vi "Toolkit Error Handling - Add Caller to API VI List.vi"(8 "error in":errorcluster) -> (0 "error out":errorcluster)   [LabVIEW 2011]
doc: "Add this VI's caller to the Toolkit API list. This is used by the Toolkit Error Handling framework to hide the call-chain of low-level support VIs."
panel:
  # "THIS VI MUST BE REENTRANT"
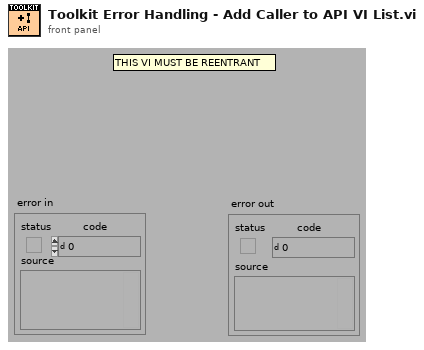
[diagram p1: front panel]
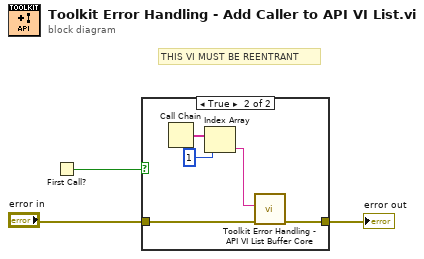
[diagram p0: block diagram]
diagram:
  # "THIS VI MUST BE REENTRANT"
  n1 = First Call?() -> (First Call?: T/F=w1:bool)
  n2 = case shown="True" w1 {
    tunnel: [w4 w9] -> w3
    tunnel: "error in" -> [w4 w8]
    frame False {
    }
    frame True {
      n3 = Call Chain() -> (call chain=w7:string[])
      n4 = Index Array(array=w7, index=1) -> (element=w5:string)
      n5 = call "Toolkit Error Handling - API VI List Buffer Core.vi"("error in (no error)"=w8, "API VI to add (\"\": get list)"=w5) -> ("error out"=w9:errorcluster)  [unwired: 8 in, 1 out]
    }
  }
  "error out" <- w3
